vi "Set Zero Mix.vi"(0 "Session Handle in":T1, 11 "error in (no error)":errorcluster) -> (4 "Session Handle out":T1, 6 "Return Code":i32, 15 "error out":errorcluster)   [LabVIEW 2015, in "Environics.lvclass"]
uses:
  Environics.lvclass
  Typedefs/Session Handle.ctl
  Environics.lvclass/Environics.ctl
  C:/TMflex/Test Fixtures/PAS Calibration/Distributed/EnvComm.dll
  EnvComm.dll
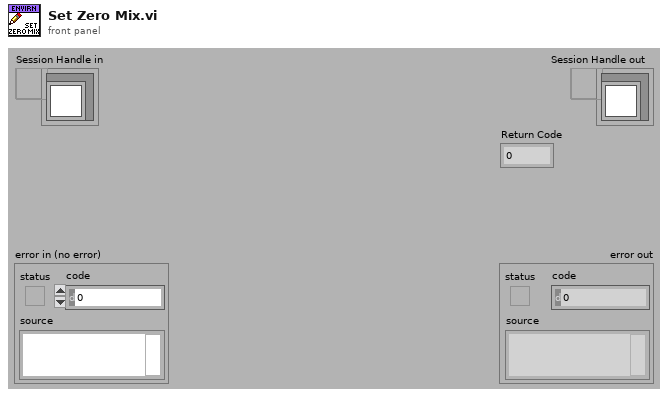
[diagram p1: front panel]
types:
  T1 = typedef "Environics.lvclass/Session Handle.ctl" = refnum<data-value>
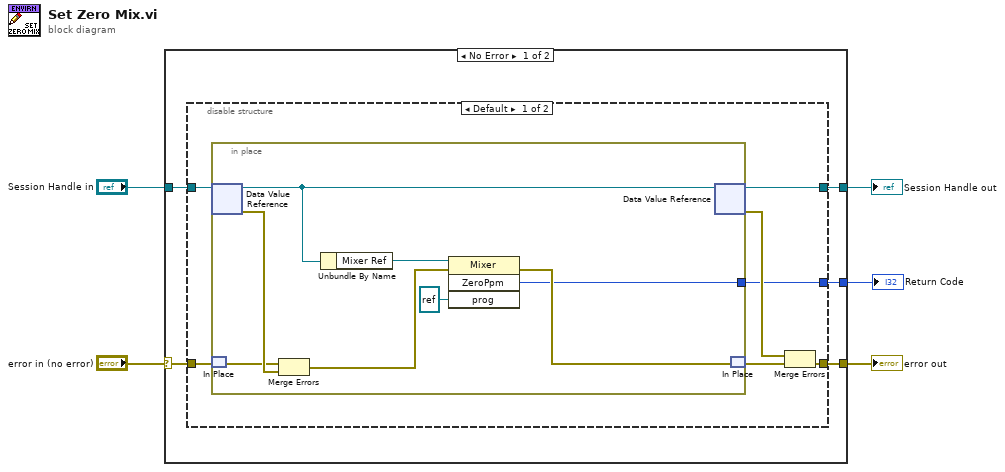
[diagram p0: block diagram]
diagram:
  n1 = case shown="No Error" "error in (no error)" {
    selector: "error in (no error)" -> [w7 w28]
    tunnel: "Session Handle in" -> [w10 w29]
    tunnel: [w9 w29] -> w4
    tunnel: [w8 w28] -> w3
    tunnel: [w6 _] -> w1
    frame No Error {
      n2 = disable-structure shown="Default" {
        disable-tunnel: w10 -> [w17 w27]
        disable-tunnel: [w16 w27] -> w9
        disable-tunnel: [w15 w26] -> w8
        disable-tunnel: w7 -> [w14 w26]
        disable-tunnel: [w11 _] -> w6
        frame condition #0 (active) {
          n3 = in-place {
            in-place-border: [w18] -> w11
            n4 = in-place-dvr #1(w17) -> (w23:refnum<class "Environics.lvclass">, w25:errorcluster)
            n5 = in-place-match #2(w14) -> (w24:errorcluster)
            n6 = Merge Errors(w24, w25) -> (w21:errorcluster)
            n7 = Unbundle By Name(w23) -> ("Mixer Ref"=w22:refnum<k24>)
            n8 = invoke class="Mixer" method="ZeroPpm"(reference=w22, error in=w21, "prog"=refnum<k24> refnum) -> (error out=w20:errorcluster, "ZeroPpm"=w18:i32)  [unwired: 1 in, 2 out]
            n9 = in-place-dvr #1(w23) -> (w16:T1, w12:errorcluster)
            n10 = in-place-match #2(w20) -> (w13:errorcluster)
          }
          n11 = Merge Errors(w12, w13) -> (w15:errorcluster)
        }
        frame condition #1 {
        }
      }
    }
    frame Error {
    }
  }
  "Session Handle out" <- w4
  "error out" <- w3
  "Return Code" <- w1
